vi "Get Path GUI.vi"() -> ()   [LabVIEW 2013, in "Data.PGSQL.lvclass"]
uses:
  Data.PGSQL.lvclass
panel:
  out "path_to_selected_column":string="llab_038:d001(TEST_TABLE--new_stuff(hippos))"
  out "selected_table":string="TEST_TABLE"
  in  "columns_list":i32(listbox)=1
  in  "tables_list":i32(listbox)=34
  in  "STOP":bool
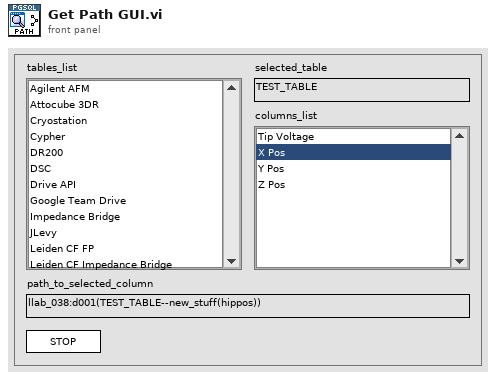
[diagram p1: front panel]
types:
  T1 = enum32{"Invalid", "Standard", "Closed", "Hidden", "Minimized", "Maximized"}
  T2 = enum32{"invalid app kind", "Development System", "Run Time System", "Student Edition", "Embedded LabVIEW", "Evaluation", "Custom"}
  T3 = cluster{"Current VI Reference":refnum<vi>, "Close Panel on Exit?":bool}
  T4 = cluster{"Core":cluster{"Current VI Reference":refnum<vi>, "Close Panel on Exit?":bool}, "Data.PG":refnum<class "Data.PGSQL.lvclass">, "table names":string[], "table paths":string[], "column names":string[], "column units":string[], "column paths":string[], "new table name":string, "new column name":string, "new column data type":string, "new column units":string, "selected table":string, "selected column":string, "selected table path":string, "selected column path":string, "max points":i32, "selected column units":string}
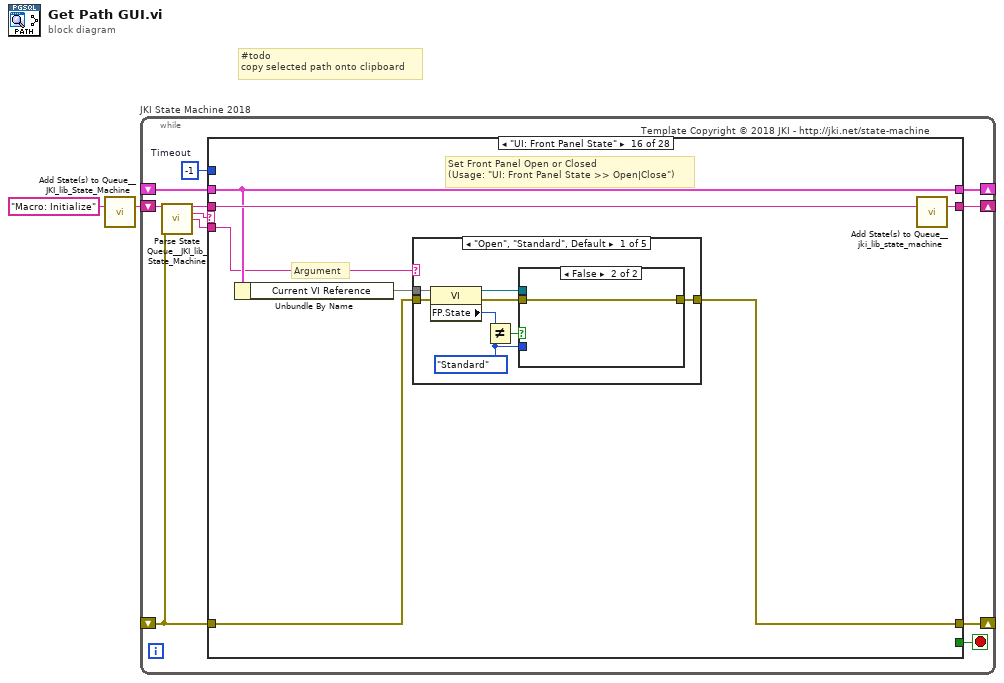
[diagram p0: block diagram]
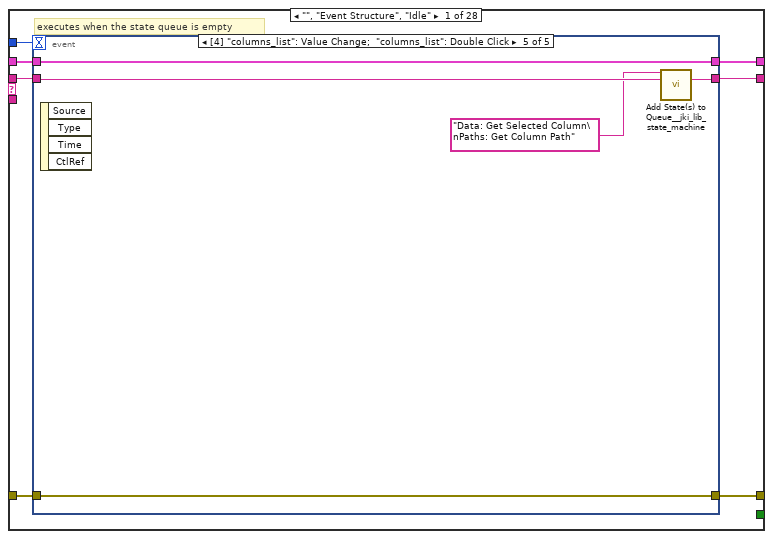
[diagram p2: hidden frame]
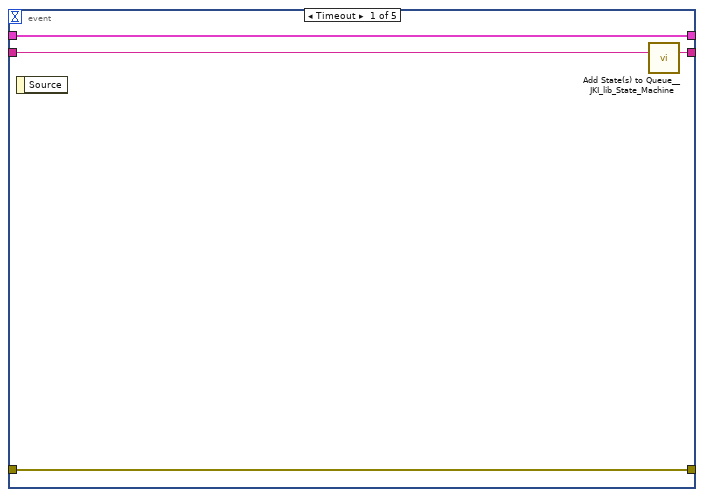
[diagram p3: hidden frame]
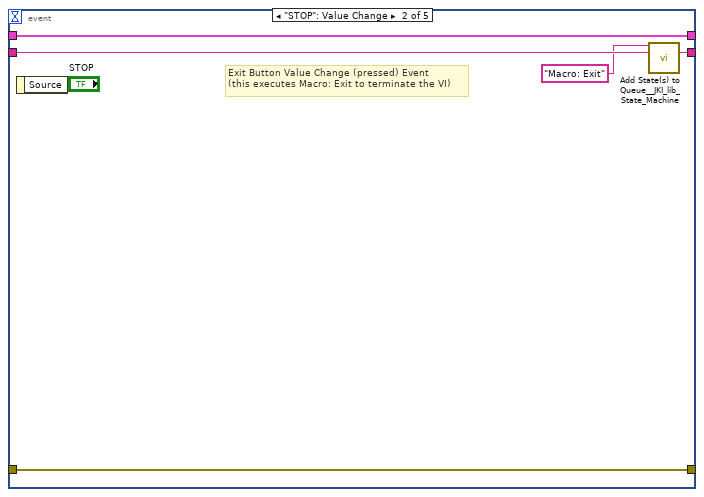
[diagram p4: hidden frame]
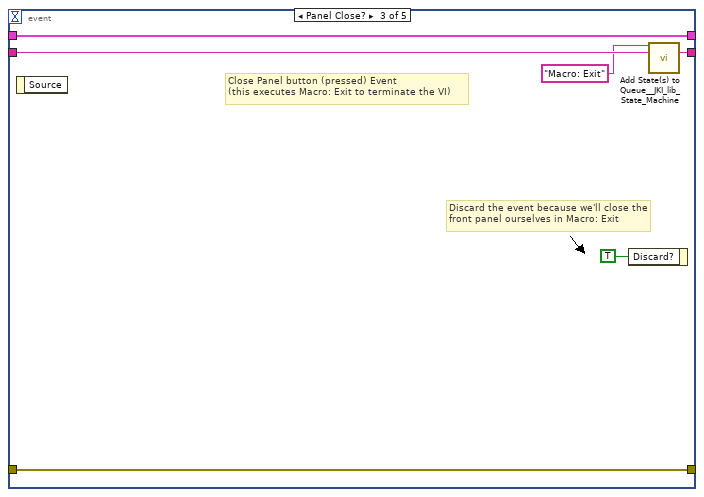
[diagram p5: hidden frame]
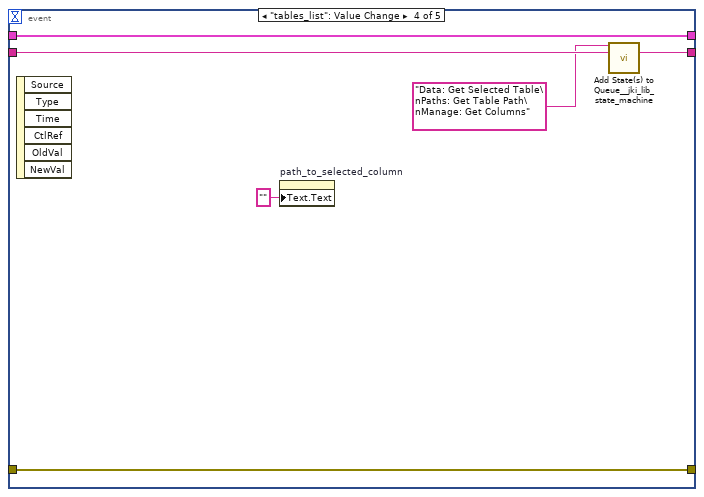
[diagram p6: hidden frame]
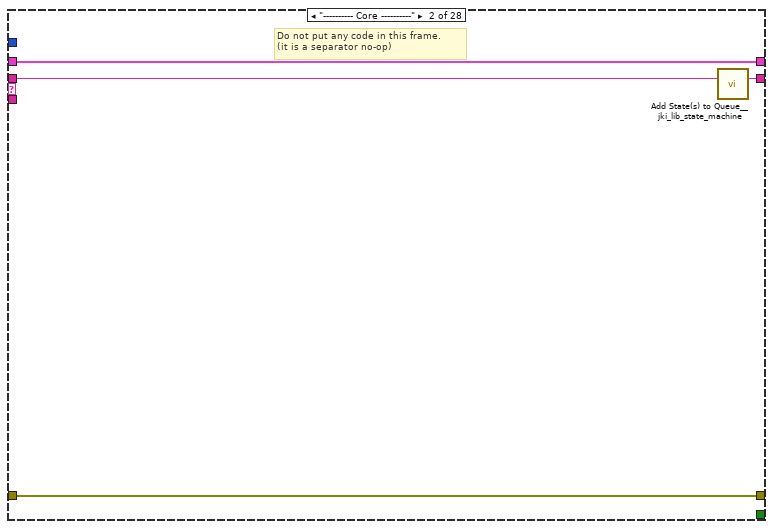
[diagram p7: hidden frame]
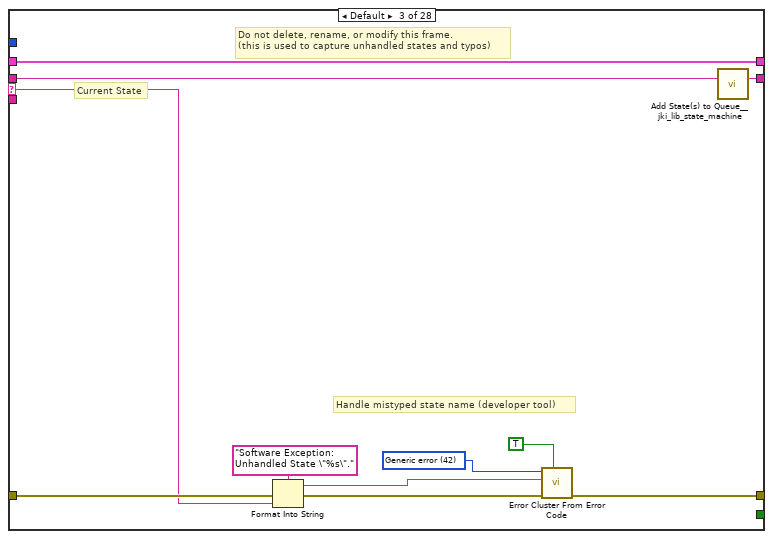
[diagram p8: hidden frame]
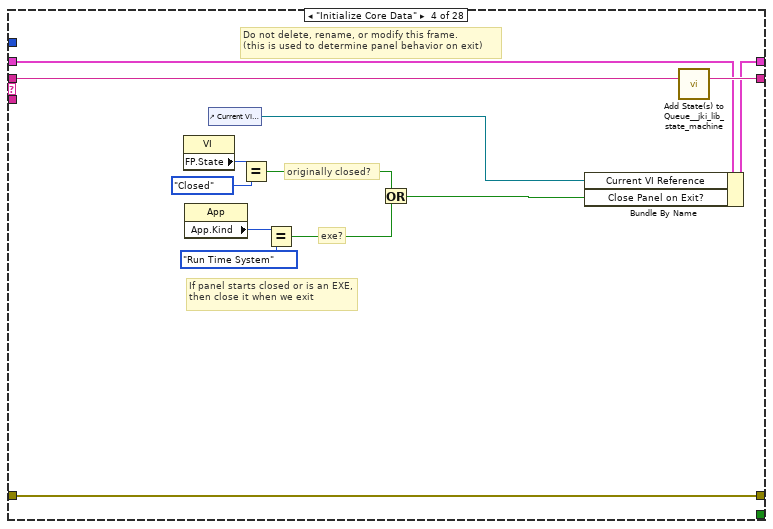
[diagram p9: hidden frame]
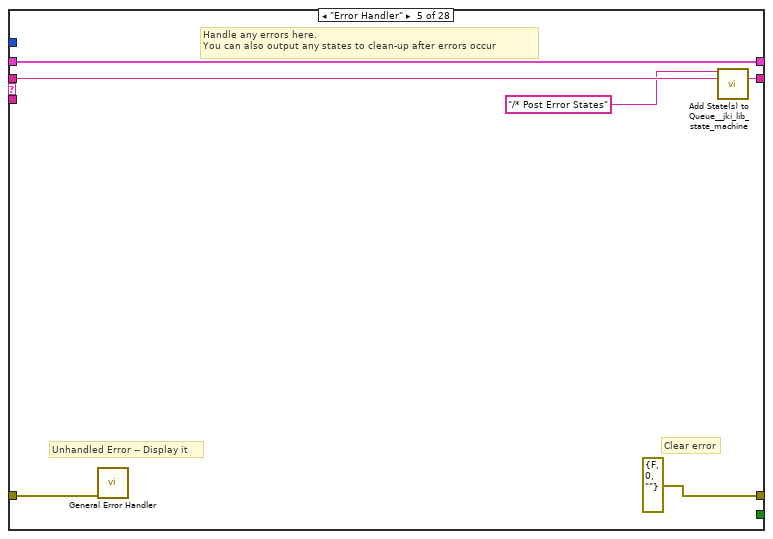
[diagram p10: hidden frame]
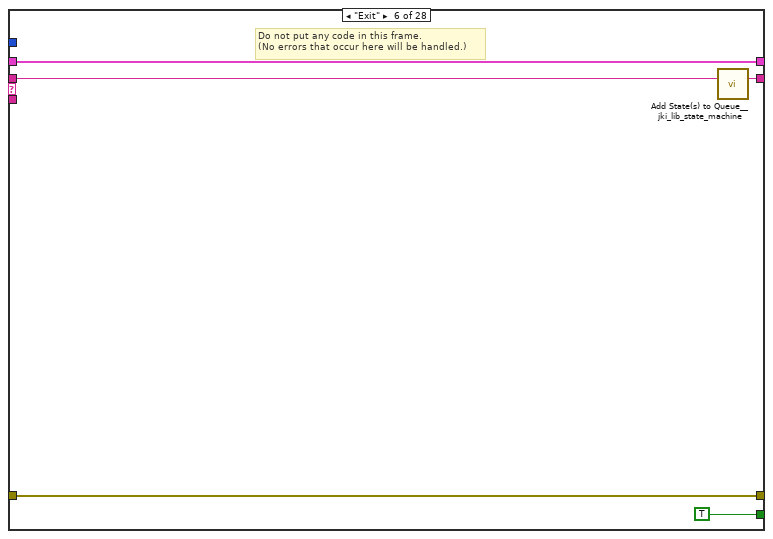
[diagram p11: hidden frame]
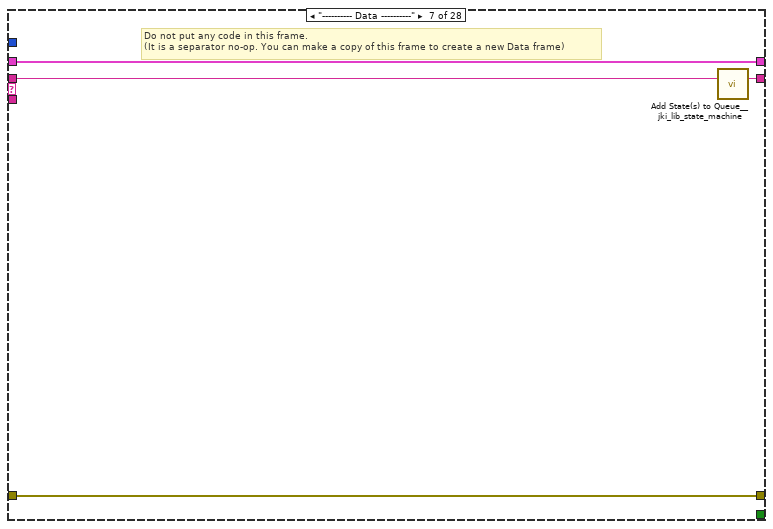
[diagram p12: hidden frame]
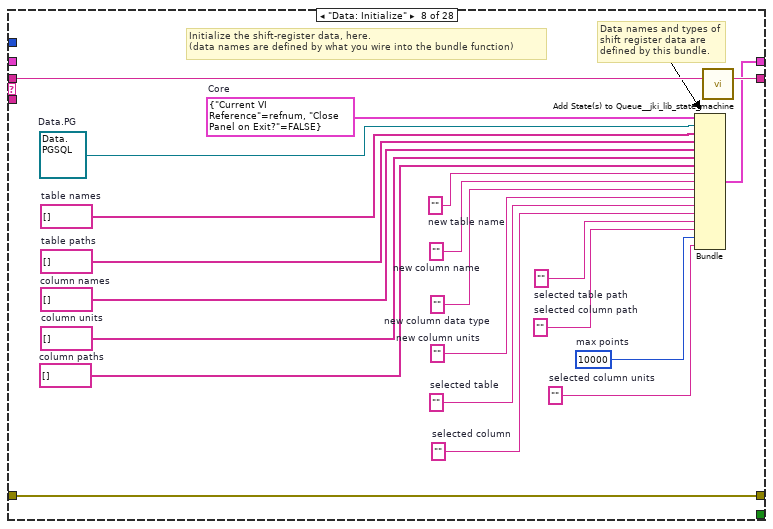
[diagram p13: hidden frame]
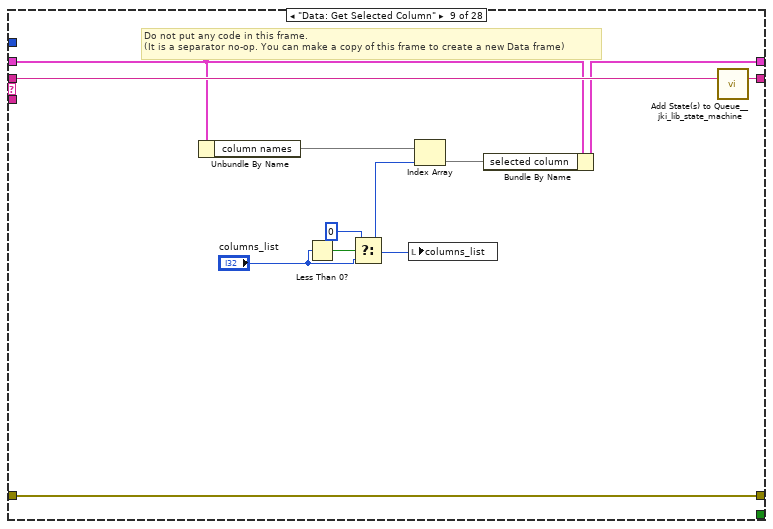
[diagram p14: hidden frame]
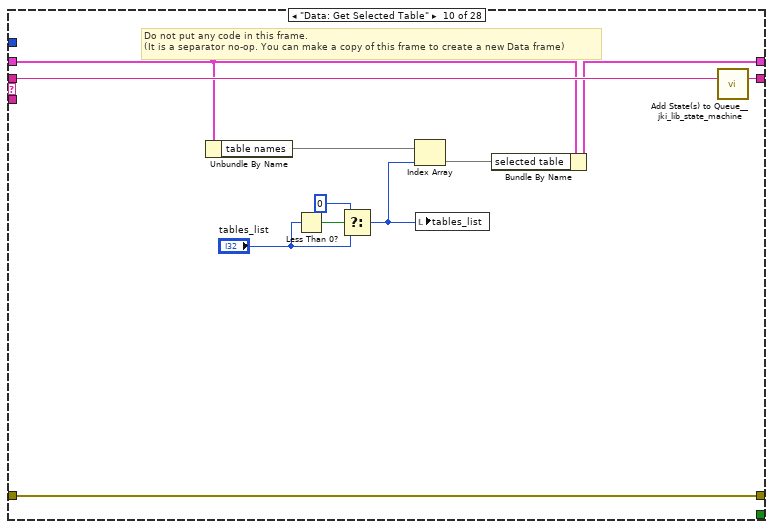
[diagram p15: hidden frame]
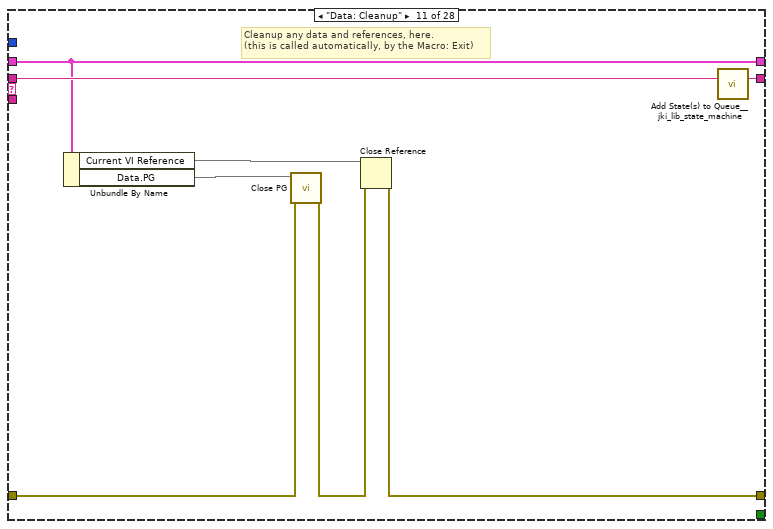
[diagram p16: hidden frame]
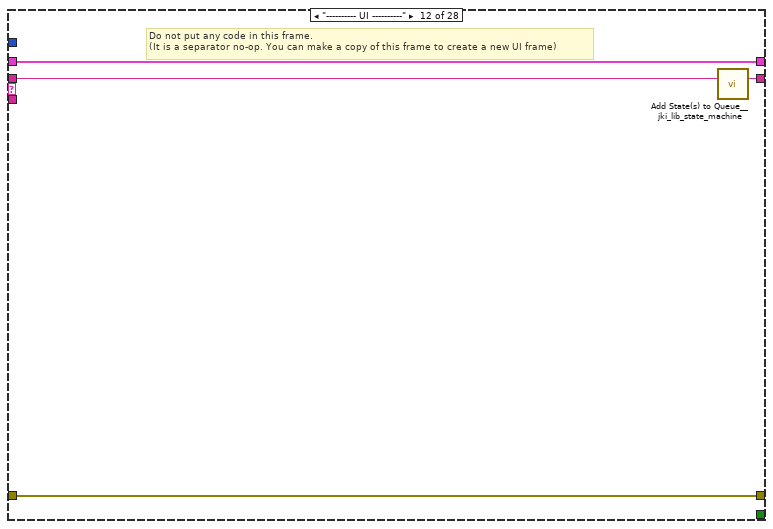
[diagram p17: hidden frame]
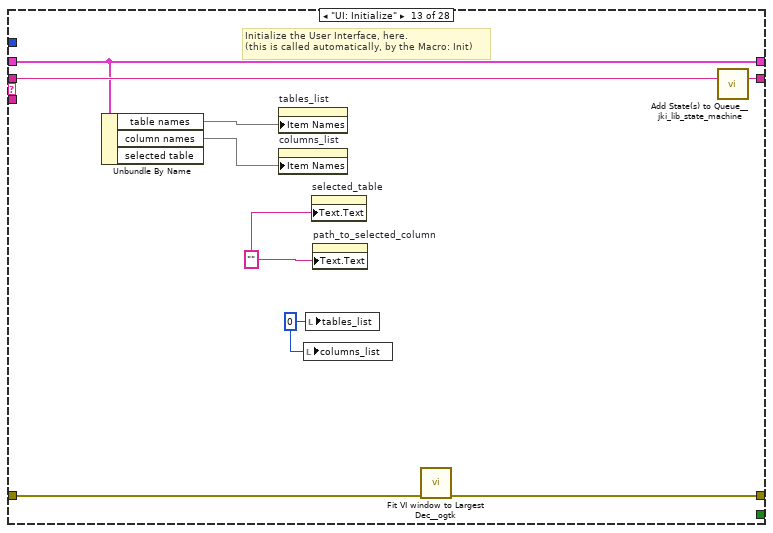
[diagram p18: hidden frame]
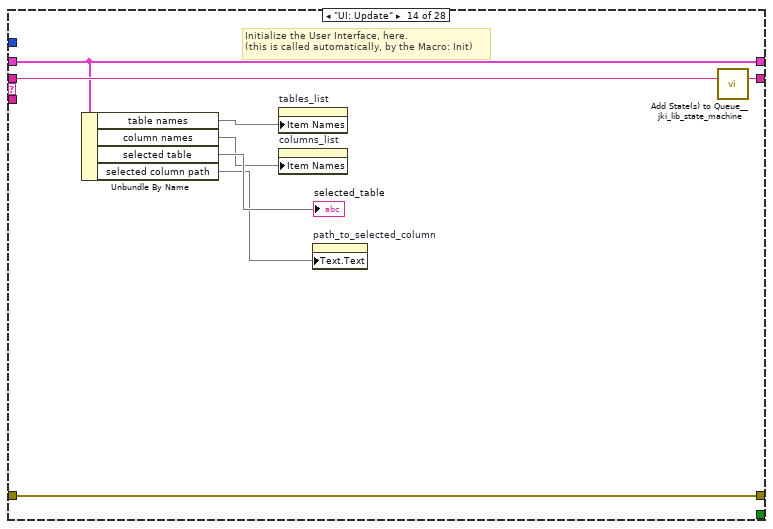
[diagram p19: hidden frame]
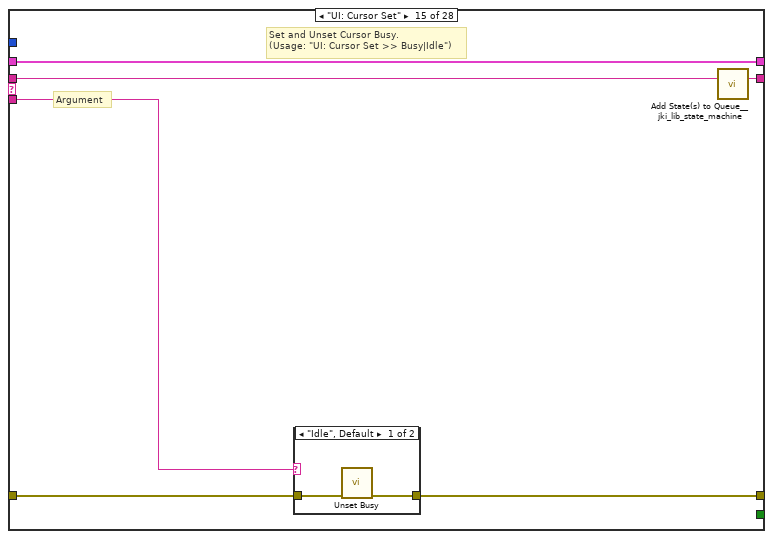
[diagram p20: hidden frame]
diagram:
  # "#todo\ncopy selected path onto clipboard"
  n1 = call <vilib>:"Add State(s) to Queue__JKI_lib_State_Machine.vi"("State(s) in (\"\")"="Macro: Initialize") -> ("States Out"=w2:string)  [unwired: 14 in]
  n2 = while "JKI State Machine 2018" {
    shift-right: [w6] -> _
    shift-left: _ -> [w5]
    shift-right: [w9] -> _
    shift-left: _ -> [w3]
    shift-right: [w8] -> _
    shift-left: w2 -> [w10]
    stop <- w7 stop-if-true
    w4 = -1  # Timeout
    # "Template Copyright © 2018 JKI - http://jki.net/state-machine"
    n3 = call <vilib>:"Parse State Queue__JKI_lib_State_Machine.vi"("State Queue"=w10, "Error In (no error)"=w3) -> ("Remaining States"=w12:string, "Current State"=w13:string, "Arguments"=w11:string)  [unwired: 11 in]
    n4 = case shown="\"UI: Front Panel State\"" w13 {
      selector: w13 -> [_ _ w51 _ _ _ _ _ _ _ _ _ _ _ _ _ _ _ _ _ _ _ _ _ _ _ _ _]
      tunnel: w12 -> [w20 w50 w55 w74 w80 w85 w89 w110 w121 w132 w140 w144 w153 w161 w167 w178 w247 w252 w262 w266 w275 w288 w292 w300 w306 w310 w319 w333]
      tunnel: w11 -> [_ _ _ _ _ _ _ _ _ _ _ _ _ _ w162 w172 _ _ _ _ _ _ _ _ _ _ _ _]
      tunnel: w5 -> [w18 w47 w53 w67 w77 w83 w86 _ w116 w127 w133 w141 w149 w158 w165 w174 w244 w249 w259 w263 w271 w280 w289 w294 w304 w307 w315 w320]
      tunnel: [w17 w48 w57 w71 errorcluster {"status"=FALSE, "code"=0, "source"=""} ("error out") w82 w87 w107 w119 w130 w134 w142 w148 w157 w163 w175 w245 w250 w260 w264 w269 w282 w290 w295 w301 w308 w312 w328] -> w9
      tunnel: w3 -> [w16 w48 w56 w71 w76 w82 w87 w107 w119 w130 w136 w142 w147 w157 w164 w176 w245 w250 w260 w264 w270 w283 w290 w296 w302 w308 w313 w329]
      tunnel: [w19 w49 w54 w73 w79 w84 w88 w109 w120 w131 w139 w143 w152 w160 w166 w177 w246 w251 w261 w265 w274 w287 w291 w299 w305 w309 w318 w332] -> w8
      tunnel: [_ _ _ _ _ TRUE _ _ _ _ _ _ _ _ _ _ _ _ _ _ _ _ _ _ _ _ _ _] -> w7
      tunnel: [w15 w47 w53 w72 w77 w83 w86 w108 w115 w126 w133 w141 w149 w158 w165 w174 w244 w249 w259 w263 w272 w281 w289 w293 w304 w307 w311 w330] -> w6
      tunnel: w4 -> [w14 _ _ _ _ _ _ _ _ _ _ _ _ _ _ _ _ _ _ _ _ _ _ _ _ _ _ _]
      frame "", "Event Structure", "Idle" {
        # "executes when the state queue is empty"
        n5 = event shown="[4] \"columns_list\": Value Change;  \"columns_list\": Double Click" {
          selector: _ -> [_ _ _ _ _]
          dyn-events: _ -> [_ _ _ _ _]
          timeout: w14 -> [_ _ _ _ _]
          tunnel: w20 -> [w24 w29 w35 w39 w45]
          tunnel: [w23 w28 w34 w40 w46] -> w19
          tunnel: w18 -> [w21 w26 w32 w36 w42]
          tunnel: [w22 w27 w33 w41 w43] -> w17
          tunnel: w16 -> [w22 w27 w33 w41 w43]
          tunnel: [w21 w26 w32 w36 w42] -> w15
          event Timeout {
            n6 = event-data() -> ()  [unwired: 1 in, 1 out]
            n7 = call <vilib>:"Add State(s) to Queue__JKI_lib_State_Machine.vi"("State(s) in (\"\")"=w24) -> ("States Out"=w23:string)  [unwired: 14 in]
          }
          event "STOP": Value Change {
            # "Exit Button Value Change (pressed) Event\n(this executes Macro: Exit to terminate the VI)"
            n8 = event-data() -> ()  [unwired: 1 in, 1 out]
            n9 = call <vilib>:"Add State(s) to Queue__JKI_lib_State_Machine.vi"("State(s) in Front (\"\")"="Macro: Exit", "State(s) in (\"\")"=w29) -> ("States Out"=w28:string)  [unwired: 13 in]
          }
          event Panel Close? {
            # "Discard the event because we'll close the front panel ourselves in Macro: Exit"
            # "Close Panel button (pressed) Event\n(this executes Macro: Exit to terminate the VI)"
            n10 = event-data() -> ()  [unwired: 1 in, 1 out]
            n11 = event-data("Discard?"=TRUE) -> ()  [unwired: 1 in, 1 out]
            n12 = call <vilib>:"Add State(s) to Queue__JKI_lib_State_Machine.vi"("State(s) in Front (\"\")"="Macro: Exit", "State(s) in (\"\")"=w35) -> ("States Out"=w34:string)  [unwired: 13 in]
          }
          event "tables_list": Value Change {
            n13 = event-data() -> ()  [unwired: 1 in, 6 out]
            n14 = property on="path_to_selected_column" class="Str"("Text.Text"="") -> ()  [unwired: 2 in, 2 out]
            n15 = call <vilib>:"Add State(s) to Queue__jki_lib_state_machine.vi"("State(s) in Front (\"\")"="Data: Get Selected Table\nPaths: Get Table Path\nManage: Get Columns" ("State(s) in Front (\"\")"), "State(s) in (\"\")"=w39) -> ("States Out"=w40:string)  [unwired: 13 in]
          }
          event "columns_list": Value Change; "columns_list": Double Click {
            n16 = event-data() -> ()  [unwired: 1 in, 4 out]
            n17 = call <vilib>:"Add State(s) to Queue__jki_lib_state_machine.vi"("State(s) in Front (\"\")"="Data: Get Selected Column\nPaths: Get Column Path", "State(s) in (\"\")"=w45) -> ("States Out"=w46:string)  [unwired: 13 in]
          }
        }
      }
      frame "---------- Core ----------" {
        # "Do not put any code in this frame.\n(it is a separator no-op)"
        n18 = call <vilib>:"Add State(s) to Queue__jki_lib_state_machine.vi"("State(s) in (\"\")"=w50) -> ("States Out"=w49:string)  [unwired: 14 in]
      }
      frame Default {
        w60 = 42 items=["No error", "Argument error", "Memory is full", "Out of zone", "End of file", "File already open", "Generic file I/O error", "File not found", "File permission error", "Disk is full", "Duplicate path", "Too many files open", "System feature not enabled", "Resource file not found", "Cannot add resource", "Resource not found", "Image not found", "Image memory error", "Pen does not exist", "Config type invalid", "Config token not found", "Config parse error", "Config memory error", "Bad external code format", "Bad external code offset", "External code not present", "Null window", "Destroy window error", "Null menu", "Print aborted", "Bad print record", "Print driver error", "Windows error during printing", "Memory error during printing", "Print dialog error", "Generic print error", "Invalid device refnum", "Device not found", "Device parameter error", "Device unit error", "Cannot open device", "Device call aborted", "Generic error", "Cancelled by user", "Object ID too low", "Object ID too high", "Object not in heap", "Unknown heap", "Unknown object (invalid DefProc)", "Unknown object (DefProc not in table)", "Message out of range", "Invalid (null) method", "Unknown message", "Manager call not supported", "Bad address", "Network operation in progress", "Network operation timed out", "Connection is busy", "Network attribute not supported", "Network error", "Address in use", "System out of memory", "Connection aborted", "Connection refused", "Not connected", "Already connected", "Connection closed", "Initialization error (interapplication manager)", "Bad occurrence", "Wait on unbound occurrence handler", "Occurrence queue overflow", "Datalog type conflict", "Unused", "Unrecognized type (interapplication manager)", "Memory corrupt", "Failed to make temporary DLL", "Old CIN version", "Drag socket not found", "Failed to load drop-object", "Failed to register OLE object", "Failed to release OLE object", "Format specifier type mismatch", "Unknown format specifier", "Too few format specifiers", "Too many format specifiers", "Scan failed", "Newer CIN version", "Error converting to variant", "Runtime menu error", "Password tampered", "Variant attribute not found", "Incompatible variant data type", "Event data is not available", "Event Store is not present", "Occurrence is not found", "Event Queue is not created", "Event info is not available", "Refnum passed is NULL", "Error retrieving Class GUID", "Error retrieving CoClass GUID", "Error retrieving TypeLib GUID.", "Bad built application magic bytes.", "Specific driver is different from the specific driver associated with the Logical Name.", "There is no session opened to the class driver.", "Max Error", "MAX - Error with config objects", "MAX - Error loading configuration", "MAX - Group not supported"]
        # "Current State"
        # "Do not delete, rename, or modify this frame.\n(this is used to capture unhandled states and typos)"
        # "Handle mistyped state name (developer tool)"
        n19 = Format Into String(format string="Software Exception: Unhandled State \"%s\"." ("message"), error in=w56, w51) -> (resulting string=w59:string, error out=w58:errorcluster)  [unwired: 1 in]
        n20 = call <vilib>:"Error Cluster From Error Code.vi"("show call chain? (False)"=TRUE, "error in (no error)"=w58, "error message (\"\")"=w59, "error code (0)"=w60) -> ("error out"=w57:errorcluster)  [unwired: 5 in]
        n21 = call <vilib>:"Add State(s) to Queue__jki_lib_state_machine.vi"("State(s) in (\"\")"=w55) -> ("States Out"=w54:string)  [unwired: 14 in]
      }
      frame "Initialize Core Data" {
        # "Do not delete, rename, or modify this frame.\n(this is used to determine panel behavior on exit)"
        # "originally closed?"
        # "exe?"
        # "If panel starts closed or is an EXE, then close it when we exit"
        n22 = property class="VI"() -> ("FP.State"=w64:T1)  [unwired: 2 in, 2 out]
        n23 = property class="App"() -> ("App.Kind"=w70:T2)  [unwired: 2 in, 2 out]
        n24 = control-ref of="Current VI Reference"() -> (w65:refnum<vi>)
        n25 = Equal?(x=w64, y=T1."Closed" ("Front Panel Window:State")) -> (x = y?=w62:bool)
        n26 = Equal?(x=w70, y=T2."Run Time System" ("Application:Kind")) -> (x = y?=w68:bool)
        n27 = Or(x=w62, y=w68) -> (x .or. y?=w66:bool)
        n28 = Bundle By Name(cluster=w67, "Current VI Reference"=w65, "Close Panel on Exit?"=w66) -> (w72:cluster{})
        n29 = call <vilib>:"Add State(s) to Queue__jki_lib_state_machine.vi"("State(s) in (\"\")"=w74) -> ("States Out"=w73:string)  [unwired: 14 in]
      }
      frame "Error Handler" {
        # "Unhandled Error -- Display it"
        # "Handle any errors here.\nYou can also output any states to clean-up after errors occur"
        # "Clear error"
        n30 = call <vilib>:"General Error Handler.vi"("error in (no error)"=w76) -> ()  [unwired: 10 in, 5 out]
        n31 = call <vilib>:"Add State(s) to Queue__jki_lib_state_machine.vi"("State(s) in Front (\"\")"="/* Post Error States", "State(s) in (\"\")"=w80) -> ("States Out"=w79:string)  [unwired: 13 in]
      }
      frame "Exit" {
        # "Do not put any code in this frame.\n(No errors that occur here will be handled.)"
        n32 = call <vilib>:"Add State(s) to Queue__jki_lib_state_machine.vi"("State(s) in (\"\")"=w85) -> ("States Out"=w84:string)  [unwired: 14 in]
      }
      frame "---------- Data ----------" {
        # "Do not put any code in this frame.\n(It is a separator no-op. You can make a copy of this frame to create a new Data frame)"
        n33 = call <vilib>:"Add State(s) to Queue__jki_lib_state_machine.vi"("State(s) in (\"\")"=w89) -> ("States Out"=w88:string)  [unwired: 14 in]
      }
      frame "Data: Initialize" {
        w90 = ""  # selected column units
        w91 = 10000  # max points
        w92 = ""  # selected column path
        w93 = ""  # selected table path
        w94 = ""  # selected column
        w95 = ""  # selected table
        w96 = ""  # new column units
        w97 = ""  # new column data type
        w98 = ""  # new column name
        w99 = ""  # new table name
        w100 = string[] []  # column paths
        w101 = string[] []  # column units
        w102 = string[] []  # column names
        w103 = string[] []  # table paths
        w104 = string[] []  # table names
        w105 = refnum<class "Data.PGSQL.lvclass"> refnum  # Data.PG
        w106 = T3 {"Current VI Reference"=refnum, "Close Panel on Exit?"=FALSE}  # Core
        # "Data names and types of shift register data are defined by this bundle."
        # "Initialize the shift-register data, here.\n(data names are defined by what you wire into the bundle function)"
        n34 = Bundle("Core"=w106, "Data.PG"=w105, "table names"=w104, "table paths"=w103, "column names"=w102, "column units"=w101, "column paths"=w100, "new table name"=w99, "new column name"=w98, "new column data type"=w97, "new column units"=w96, "selected table"=w95, "selected column"=w94, "selected table path"=w93, "selected column path"=w92, "max points"=w91, "selected column units"=w90) -> (w108:T4)  [unwired: 1 in]
        n35 = call <vilib>:"Add State(s) to Queue__jki_lib_state_machine.vi"("State(s) in (\"\")"=w110) -> ("States Out"=w109:string)  [unwired: 14 in]
      }
      frame "Data: Get Selected Column" {
        # "Do not put any code in this frame.\n(It is a separator no-op. You can make a copy of this frame to create a new Data frame)"
        n36 = Unbundle By Name(w116) -> ("column names"=w118)
        n37 = Less Than 0?(x="columns_list") -> (x < 0?=w114:bool)
        n38 = Select(t=0, s=w114, f="columns_list") -> (s? t:f=w111:i32)
        n39 = local write "columns_list"(w111) -> ()
        n40 = Index Array(array=w118, index=w111) -> (element=w117)
        n41 = Bundle By Name(cluster=w116, "selected column"=w117) -> (w115:cluster{})
        n42 = call <vilib>:"Add State(s) to Queue__jki_lib_state_machine.vi"("State(s) in (\"\")"=w121) -> ("States Out"=w120:string)  [unwired: 14 in]
      }
      frame "Data: Get Selected Table" {
        # "Do not put any code in this frame.\n(It is a separator no-op. You can make a copy of this frame to create a new Data frame)"
        n43 = Unbundle By Name(w127) -> ("table names"=w129)
        n44 = Less Than 0?(x="tables_list") -> (x < 0?=w125:bool)
        n45 = Select(t=0, s=w125, f="tables_list") -> (s? t:f=w123:i32)
        n46 = Index Array(array=w129, index=w123) -> (element=w128)
        n47 = local write "tables_list"(w123) -> ()
        n48 = Bundle By Name(cluster=w127, "selected table"=w128) -> (w126:cluster{})
        n49 = call <vilib>:"Add State(s) to Queue__jki_lib_state_machine.vi"("State(s) in (\"\")"=w132) -> ("States Out"=w131:string)  [unwired: 14 in]
      }
      frame "Data: Cleanup" {
        # "Cleanup any data and references, here.\n(this is called automatically, by the Macro: Exit)"
        n50 = Unbundle By Name(w133) -> ("Current VI Reference"=w138, "Data.PG"=w137)
        n51 = call-dynamic "Close PG.vi"("error in (no error)"=w136, "Data.PG in"=w137) -> ("error out"=w135:errorcluster)  [unwired: 8 in, 1 out]
        n52 = Close Reference(reference=w138, error in (no error)=w135) -> (error out=w134:errorcluster)
        n53 = call <vilib>:"Add State(s) to Queue__jki_lib_state_machine.vi"("State(s) in (\"\")"=w140) -> ("States Out"=w139:string)  [unwired: 14 in]
      }
      frame "---------- UI ----------" {
        # "Do not put any code in this frame.\n(It is a separator no-op. You can make a copy of this frame to create a new UI frame)"
        n54 = call <vilib>:"Add State(s) to Queue__jki_lib_state_machine.vi"("State(s) in (\"\")"=w144) -> ("States Out"=w143:string)  [unwired: 14 in]
      }
      frame "UI: Initialize" {
        w146 = 0 ("tables_list")
        w145 = "" ("Text.Text")
        # "Initialize the User Interface, here.\n(this is called automatically, by the Macro: Init)"
        n55 = Unbundle By Name(w149) -> ("table names"=w151, "column names"=w150)  [unwired: 1 out]
        n56 = property on="tables_list" class="LstBox (strict)"("Item Names"=w151) -> ()  [unwired: 2 in, 2 out]
        n57 = property on="columns_list" class="LstBox (strict)"("Item Names"=w150) -> ()  [unwired: 2 in, 2 out]
        n58 = local write "columns_list"(w146) -> ()
        n59 = local write "tables_list"(w146) -> ()
        n60 = property on="selected_table" class="Str"("Text.Text"=w145) -> ()  [unwired: 2 in, 2 out]
        n61 = property on="path_to_selected_column" class="Str"("Text.Text"=w145) -> ()  [unwired: 2 in, 2 out]
        n62 = call <userlib>:"Fit VI window to Largest Dec__ogtk.vi"("error in (no error)"=w147) -> ("error out"=w148:errorcluster)  [unwired: 5 in, 1 out]
        n63 = call <vilib>:"Add State(s) to Queue__jki_lib_state_machine.vi"("State(s) in (\"\")"=w153) -> ("States Out"=w152:string)  [unwired: 14 in]
      }
      frame "UI: Update" {
        # "Initialize the User Interface, here.\n(this is called automatically, by the Macro: Init)"
        n64 = Unbundle By Name(w158) -> ("table names"=w159, "column names"=w155, "selected table"=→"selected_table", "selected column path"=w154)
        n65 = property on="tables_list" class="LstBox (strict)"("Item Names"=w159) -> ()  [unwired: 2 in, 2 out]
        n66 = property on="columns_list" class="LstBox (strict)"("Item Names"=w155) -> ()  [unwired: 2 in, 2 out]
        n67 = property on="path_to_selected_column" class="Str"("Text.Text"=w154) -> ()  [unwired: 2 in, 2 out]
        n68 = call <vilib>:"Add State(s) to Queue__jki_lib_state_machine.vi"("State(s) in (\"\")"=w161) -> ("States Out"=w160:string)  [unwired: 14 in]
      }
      frame "UI: Cursor Set" {
        # "Argument"
        # "Set and Unset Cursor Busy.\n(Usage: \"UI: Cursor Set >> Busy|Idle\")"
        n69 = case shown="\"Idle\", Default" w162 {
          tunnel: w164 -> [w169 w171]
          tunnel: [w168 w170] -> w163
          frame "Idle", Default {
            n70 = call <vilib>:"Unset Busy.vi"("error in (no error)"=w169) -> ("error out"=w168:errorcluster)  [unwired: 10 in]
          }
          frame "Busy" {
            n71 = call <vilib>:"Set Busy.vi"("error in (no error)"=w171) -> ("error out"=w170:errorcluster)  [unwired: 9 in, 1 out]
          }
        }
        n72 = call <vilib>:"Add State(s) to Queue__jki_lib_state_machine.vi"("State(s) in (\"\")"=w167) -> ("States Out"=w166:string)  [unwired: 14 in]
      }
      frame "UI: Front Panel State" {
        # "Argument"
        # "Set Front Panel Open or Closed\n(Usage: \"UI: Front Panel State >> Open|Close\")"
        n73 = Unbundle By Name(w174) -> ("Current VI Reference"=w173)
        n74 = case shown="\"Open\", \"Standard\", Default" w172 {
          tunnel: w176 -> [w184 w199 w210 w223 w236]
          tunnel: [w186 w200 w212 w225 w238] -> w175
          tunnel: w173 -> [w185 w197 w211 w224 w237]
          frame "Open", "Standard", Default {
            w179 = T1."Standard" ("State")
            n75 = property class="VI"(reference=w185, error in=w184) -> (reference out=w182:refnum<vi>, error out=w183:errorcluster, "FP.State"=w181:T1)
            n76 = Not Equal?(x=w181, y=w179) -> (x != y?=w180:bool)
            n77 = case shown="False" w180 {
              tunnel: [w190 w192] -> w186
              tunnel: w183 -> [w189 w192]
              tunnel: w182 -> [w188 _]
              tunnel: w179 -> [w187 _]
              frame True {
                n78 = invoke class="VI" method="FP.Open"(reference=w188, error in=w189, "Activate"=TRUE, "State"=w187) -> (error out=w190:errorcluster)  [unwired: 1 in, 4 out]
              }
              frame False {
              }
            }
          }
          frame "Close", "Closed" {
            n79 = property class="VI"(reference=w197, error in=w199) -> (reference out=w196:refnum<vi>, error out=w198:errorcluster, "FP.State"=w194:T1)
            n80 = Not Equal?(x=w194, y=T1."Closed" ("Front Panel Window:State")) -> (x != y?=w193:bool)
            n81 = case shown="True" w193 {
              tunnel: [w201 w204] -> w200
              tunnel: w198 -> [w201 w203]
              tunnel: w196 -> [_ w202]
              frame False {
              }
              frame True {
                n82 = invoke class="VI" method="FP.Close"(reference=w202, error in=w203) -> (error out=w204:errorcluster)  [unwired: 1 in, 2 out]
              }
            }
          }
          frame "Hidden", "Hide" {
            w205 = T1."Hidden" ("State")
            n83 = property class="VI"(reference=w211, error in=w210) -> (reference out=w208:refnum<vi>, error out=w209:errorcluster, "FP.State"=w207:T1)
            n84 = Not Equal?(x=w207, y=w205) -> (x != y?=w206:bool)
            n85 = case shown="True" w206 {
              tunnel: [w216 w217] -> w212
              tunnel: w209 -> [w215 w217]
              tunnel: w208 -> [w214 _]
              tunnel: w205 -> [w213 _]
              frame True {
                n86 = invoke class="VI" method="FP.Open"(reference=w214, error in=w215, "State"=w213) -> (error out=w216:errorcluster)  [unwired: 2 in, 4 out]
              }
              frame False {
              }
            }
          }
          frame "Minimize", "Minimized" {
            w218 = T1."Minimized" ("State")
            n87 = property class="VI"(reference=w224, error in=w223) -> (reference out=w221:refnum<vi>, error out=w222:errorcluster, "FP.State"=w220:T1)
            n88 = Not Equal?(x=w220, y=w218) -> (x != y?=w219:bool)
            n89 = case shown="True" w219 {
              tunnel: [w229 w230] -> w225
              tunnel: w222 -> [w228 w230]
              tunnel: w221 -> [w227 _]
              tunnel: w218 -> [w226 _]
              frame True {
                n90 = invoke class="VI" method="FP.Open"(reference=w227, error in=w228, "State"=w226) -> (error out=w229:errorcluster)  [unwired: 2 in, 4 out]
              }
              frame False {
              }
            }
          }
          frame "Maximize", "Maximized" {
            w231 = T1."Maximized" ("State")
            n91 = property class="VI"(reference=w237, error in=w236) -> (reference out=w234:refnum<vi>, error out=w235:errorcluster, "FP.State"=w233:T1)
            n92 = Not Equal?(x=w233, y=w231) -> (x != y?=w232:bool)
            n93 = case shown="True" w232 {
              tunnel: [w242 w243] -> w238
              tunnel: w235 -> [w241 w243]
              tunnel: w234 -> [w240 _]
              tunnel: w231 -> [w239 _]
              frame True {
                n94 = invoke class="VI" method="FP.Open"(reference=w240, error in=w241, "State"=w239) -> (error out=w242:errorcluster)  [unwired: 2 in, 4 out]
              }
              frame False {
              }
            }
          }
        }
        n95 = call <vilib>:"Add State(s) to Queue__jki_lib_state_machine.vi"("State(s) in (\"\")"=w178) -> ("States Out"=w177:string)  [unwired: 14 in]
      }
      frame "---------- Macro ----------" {
        # "Do not put any code in this frame.\n(It is a separator no-op. You can make a copy of this frame to create a new Macro frame)"
        n96 = call <vilib>:"Add State(s) to Queue__jki_lib_state_machine.vi"("State(s) in (\"\")"=w247) -> ("States Out"=w246:string)  [unwired: 14 in]
      }
      frame "Macro: Initialize" {
        # "Initialization Macro\n(This is called once, when the VI starts)"
        n97 = call <vilib>:"Add State(s) to Queue__jki_lib_state_machine.vi"("State(s) in Front (\"\")"="Data: Initialize\nInitialize Core Data\nUI: Initialize\nUI: Front Panel State >> Open\n\nConnection: Open\nManage: Get Tables\nUI: Update\n\nData: Get Selected Table\nPaths: Get Table Path\n\nManage: Get Columns\nUI: Update\nData: Get Selected Column\n\nPaths: Get Column Path", "State(s) in (\"\")"=w252) -> ("States Out"=w251:string)  [unwired: 13 in]
      }
      frame "Macro: Exit" {
        # "Exit Macro\n(This is called once, when the VI exits)"
        n98 = Unbundle By Name(w259) -> ("Close Panel on Exit?"=w258)
        n99 = Select(t="UI: Front Panel State >> Close", s=w258, f="") -> (s? t:f=w255:string)
        n100 = call <vilib>:"Add State(s) to Queue__jki_lib_state_machine.vi"("State(s) in (\"\")"=w255, "State(s) at Back (\"\")"="Data: Cleanup\nConnection: Close\nExit") -> ("States Out"=w253:string)  [unwired: 13 in]
        n101 = call <vilib>:"Add State(s) to Queue__jki_lib_state_machine.vi"("State(s) in Front (\"\")"=w253, "State(s) in (\"\")"=w262) -> ("States Out"=w261:string)  [unwired: 13 in]
      }
      frame "---------- Manage ----------" {
        # "Template Separator\n(You can make a copy of, or modify, this frame)"
        n102 = call <vilib>:"Add State(s) to Queue__jki_lib_state_machine.vi"("State(s) in (\"\")"=w266) -> ("States Out"=w265:string)  [unwired: 14 in]
      }
      frame "Manage: Get Tables" {
        # "Your code here.\n(You can make a copy of, or modify, this frame)"
        n103 = Unbundle By Name(w271) -> ("Data.PG"=w273)
        n104 = call "Get Tables.vi"("error in (no error)"=w270, "Data.PG"=w273) -> ("error out"=w269:errorcluster, "Table Paths"=w267:string[], "Table Names"=w268:string[])  [unwired: 6 in, 1 out]
        n105 = Bundle By Name(cluster=w271, "table names"=w268, "table paths"=w267) -> (w272:cluster{})
        n106 = call <vilib>:"Add State(s) to Queue__jki_lib_state_machine.vi"("State(s) in (\"\")"=w275) -> ("States Out"=w274:string)  [unwired: 14 in]
      }
      frame "Manage: Get Columns" {
        # "Your code here.\n(You can make a copy of, or modify, this frame)"
        n107 = Unbundle By Name(w280) -> ("Data.PG"=w286, "selected table path"=w285)
        n108 = call "Get Columns.vi"("error in (no error)"=w283, "selected table path"=w285, "Data.PG in"=w286) -> ("error out"=w282:errorcluster, "Column Paths"=w278:string[], "Column Names"=w279:string[], "Data.PG out"=w276:refnum<class "Data.PGSQL.lvclass">, "Column Units"=w277:string[])  [unwired: 4 in]
        n109 = Bundle By Name(cluster=w280, "Data.PG"=w276, "column names"=w279, "column paths"=w278, "column units"=w277) -> (w281:cluster{})
        n110 = call <vilib>:"Add State(s) to Queue__jki_lib_state_machine.vi"("State(s) in Front (\"\")"="UI: Update" ("State(s) in Front (\"\")"), "State(s) in (\"\")"=w288) -> ("States Out"=w287:string)  [unwired: 13 in]
      }
      frame "---------- Connection ----------" {
        # "Template Separator\n(You can make a copy of, or modify, this frame)"
        n111 = call <vilib>:"Add State(s) to Queue__jki_lib_state_machine.vi"("State(s) in (\"\")"=w292) -> ("States Out"=w291:string)  [unwired: 14 in]
      }
      frame "Connection: Open" {
        # "#todo\n- Should we call Open.vi here?\n- Should Open.vi call \"Get Connection Info\"?"
        # "Template Separator\n(You can make a copy of, or modify, this frame)"
        n112 = Unbundle By Name(w294) -> ("Data.PG"=w298)
        n113 = call "Set Connection Info.vi"("Data.PG in"=w298, "error in (no error)"=w296) -> ("Data.PG out"=w297:refnum<class "Data.PGSQL.lvclass">, "error out"=w295:errorcluster)  [unwired: 7 in]
        n114 = Bundle By Name(cluster=w294, "Data.PG"=w297) -> (w293:cluster{})
        n115 = call <vilib>:"Add State(s) to Queue__jki_lib_state_machine.vi"("State(s) in (\"\")"=w300) -> ("States Out"=w299:string)  [unwired: 14 in]
      }
      frame "Connection: Close" {
        # "Template Separator\n(You can make a copy of, or modify, this frame)"
        n116 = Unbundle By Name(w304) -> ("Data.PG"=w303)
        n117 = call-dynamic "Close PG.vi"("error in (no error)"=w302, "Data.PG in"=w303) -> ("error out"=w301:errorcluster)  [unwired: 8 in, 1 out]
        n118 = call <vilib>:"Add State(s) to Queue__jki_lib_state_machine.vi"("State(s) in (\"\")"=w306) -> ("States Out"=w305:string)  [unwired: 14 in]
      }
      frame "---------- Paths ----------" {
        # "Template Separator\n(You can make a copy of, or modify, this frame)"
        n119 = call <vilib>:"Add State(s) to Queue__jki_lib_state_machine.vi"("State(s) in (\"\")"=w310) -> ("States Out"=w309:string)  [unwired: 14 in]
      }
      frame "Paths: Get Table Path" {
        # "Template Separator\n(You can make a copy of, or modify, this frame)"
        n120 = Unbundle By Name(w315) -> ("Data.PG"=w317, "selected table"=w316)
        n121 = call "Get Table Path.vi"("error in (no error)"=w313, "Table"=w316, "Data.PG"=w317) -> ("error out"=w312:errorcluster, "Table Path"=w314:string)  [unwired: 6 in, 1 out]
        n122 = Bundle By Name(cluster=w315, "selected table path"=w314) -> (w311:cluster{})
        n123 = call <vilib>:"Add State(s) to Queue__jki_lib_state_machine.vi"("State(s) in (\"\")"=w319) -> ("States Out"=w318:string)  [unwired: 14 in]
      }
      frame "Paths: Get Column Path" {
        # "Template Separator\n(You can make a copy of, or modify, this frame)"
        n124 = Unbundle By Name(w320) -> ("Data.PG"=w331, "selected table path"=w326, "selected column"=w322, "selected table"=w323, "selected column"=w327)
        n125 = call "Get Column Path.vi"("error in (no error)"=w329, "Column"=w322, "Table path"=w326, "Data.PG in"=w331) -> ("error out"=w328:errorcluster, "Column Unit"=w325:string, "Column Path"=w324:string)  [unwired: 4 in, 1 out]
        n126 = call "Build Path.vi"("Table path"=w326, "Column path"=w324, "Table name"=w323, "Column name"=w327, "Column units"=w325) -> ("PG path"=w321:string)  [unwired: 10 in]
        "path_to_selected_column" <- w321
        n127 = Bundle By Name(cluster=w320, "selected column path"=w324, "selected column units"=w325) -> (w330:cluster{})
        n128 = invoke class="App" method="Clipboard.Write"("Param 0"=w321) -> ()  [unwired: 3 in, 4 out]
        n129 = call <vilib>:"Add State(s) to Queue__jki_lib_state_machine.vi"("State(s) in (\"\")"=w333) -> ("States Out"=w332:string)  [unwired: 14 in]
      }
    }
  }
